vi "4Pi DCM - Crop Image.vi"(9 "ROI Size":i32=3, 10 "Image Refs":T1[](array[typedef]), 11 "Input Image (U16)":u16[][](array[numeric])) -> (3 "Output Image Stack":u16[][][](array[numeric]))   [LabVIEW 2016]
uses:
  <vilib>/vision/Image Controls.llb/IMAQ Image.ctl
  Display Module/Display Module Custom Controls/ROI Descriptor.ctl
panel:
  out "ROI4":u16[][](graph)
  out "ROI3":u16[][](graph)
  out "ROI2":u16[][](graph)
  out "ROI1":u16[][](graph)
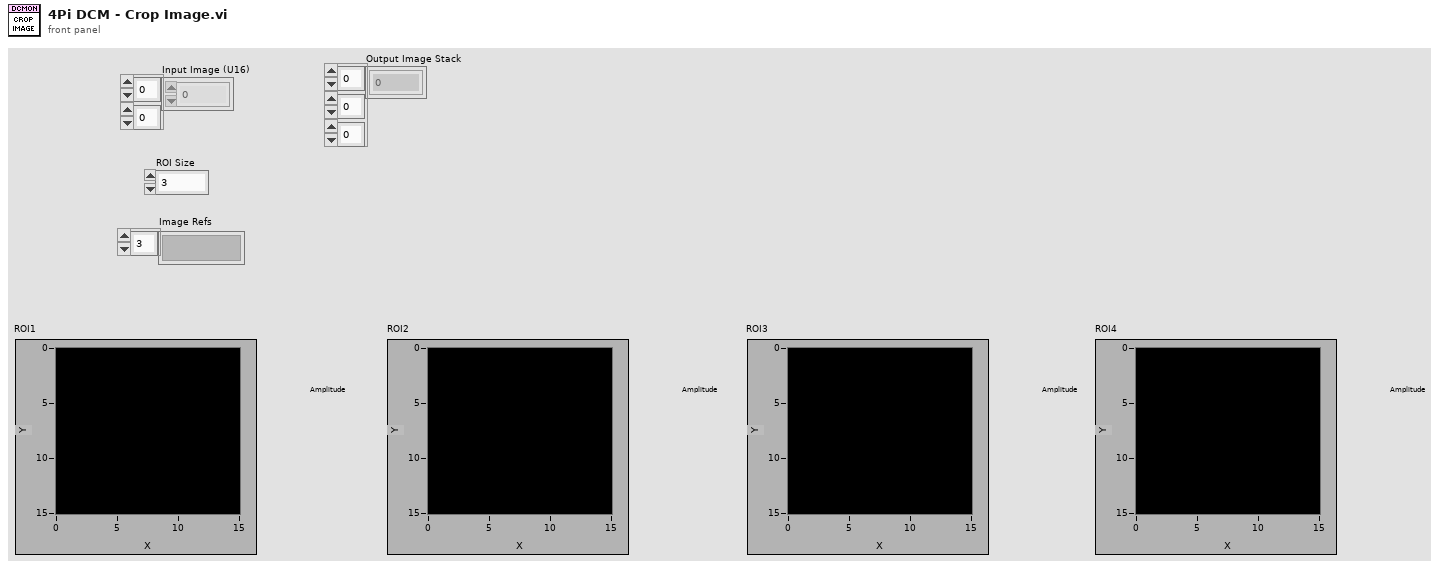
[diagram p1: front panel]
types:
  T1 = typedef "IMAQ Image.ctl" = refnum<image>
  T2 = typedef "ROI Descriptor.ctl" = cluster{"Global Rectangle":i32[], "Contours":cluster{"Contour Type":u32, "ROI Type":u32, "Points":i32[]}[]}
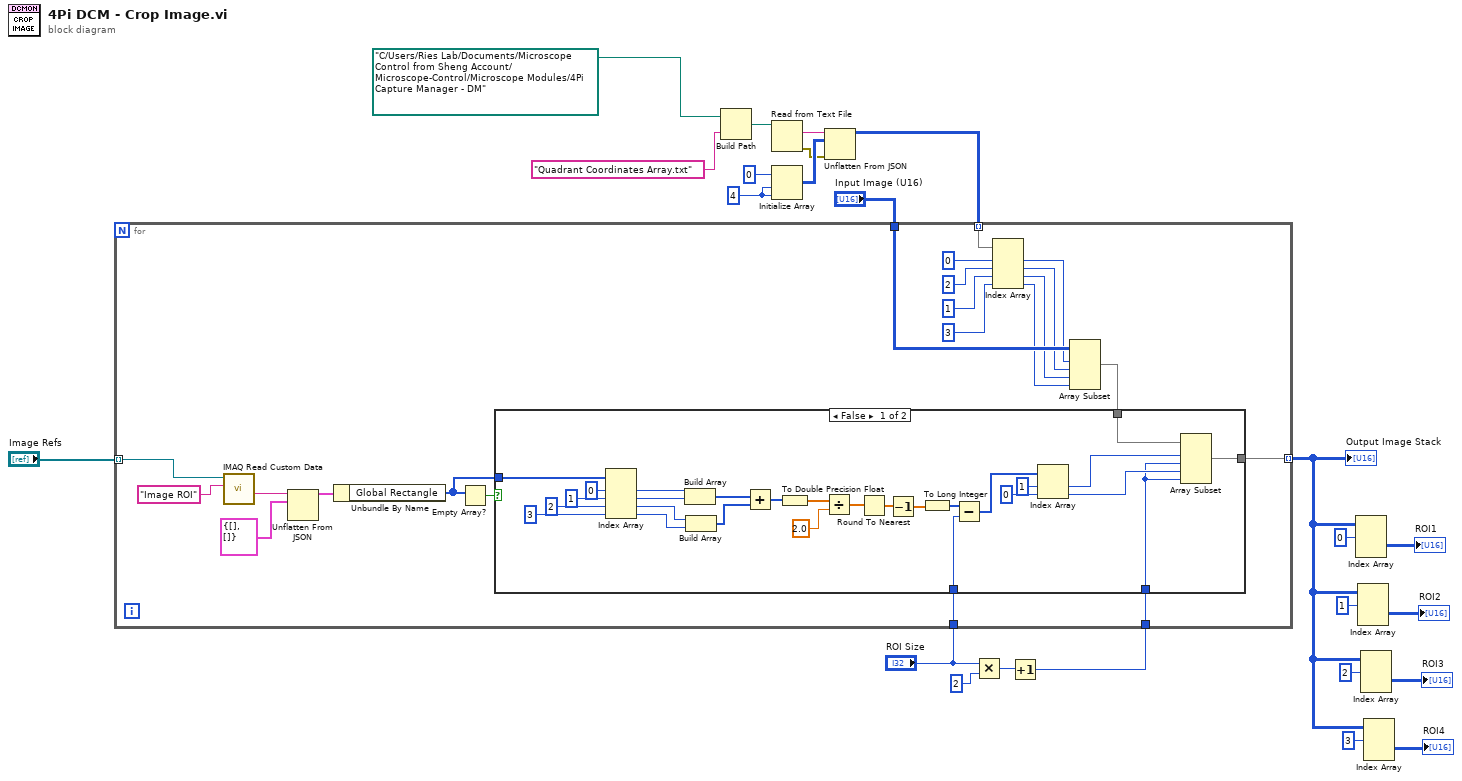
[diagram p0: block diagram]
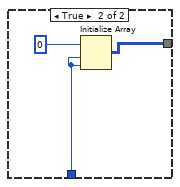
[diagram p2: hidden frame]
diagram:
  w18 = 4 ("dimension size")
  n1 = Build Path(base path=path "C:/Users/Ries Lab/Documents/Microscope Control from Sheng Account/Microscope-Control/Microscope Modules/4Pi Capture Manager - DM" ("path"), name or relative path="Quadrant Coordinates Array.txt") -> (appended path=w21:path)
  n2 = Read from Text File(file (use dialog)=w21) -> (text=w20:string, error out=w19:errorcluster)  [unwired: 3 in, 2 out]
  n3 = Initialize Array(0 ("element"), w18, w18) -> (w22:i32[][])
  n4 = Unflatten From JSON(JSON string=w20, type and defaults=w22, error in (no error)=w19) -> (value=w17:i32[][])  [unwired: 4 in, 1 out]
  n5 = Multiply(x="ROI Size", y=2) -> (x*y=w14:i32)
  n6 = Increment(x=w14) -> (x+1=w13:i32)
  n7 = for {
    tunnel: w17 -> [w45] mode=indexing
    tunnel: "Input Image (U16)" -> [w44]
    tunnel: w13 -> [w28]
    tunnel: "ROI Size" -> [w27]
    tunnel: [w26] -> w2 mode=indexing
    tunnel: "Image Refs" -> [w25] mode=indexing
    n8 = call "IMAQ Read Custom Data"("Key"="Image ROI", "Image"=w25) -> ("Custom Data Out"=w33:string)  [unwired: 7 in, 2 out]
    n9 = Unflatten From JSON(JSON string=w33, type and defaults=T2 {"Global Rectangle"=[], "Contours"=[]} ("Image ROI Descriptor")) -> (value=w31:T2)  [unwired: 5 in, 1 out]
    n10 = Unbundle By Name(w31) -> ("Global Rectangle"=w29:i32[])
    n11 = Empty Array?(array=w29) -> (empty?=w30:bool)
    n12 = Index Array(array=w45, index #1=0 ("index"), index #2=2 ("index"), index #3=1 ("index"), index #4=3 ("index")) -> (element #1=w42:i32, element #2=w41:i32, element #3=w37:i32, element #4=w36:i32)
    n13 = Array Subset(array=w44, index (row)=w42, length (row)=w41, index (col)=w37, length (col)=w36) -> (w35:u16[][])
    n14 = case shown="False" w30 {
      tunnel: w35 -> [w52 _]
      tunnel: [w51 w73] -> w26
      tunnel: w29 -> [w50 _]
      tunnel: w28 -> [w49 w74]
      tunnel: w27 -> [w48 _]
      frame False {
        n15 = Index Array(array=w50, index #1=0 ("index"), index #2=1 ("index"), index #3=2 ("index"), index #4=3 ("index")) -> (element #1=w65:i32, element #2=w64:i32, element #3=w63:i32, element #4=w62:i32)
        n16 = Build Array(w65, w64) -> (w61:i32[])
        n17 = Build Array(w63, w62) -> (w60:i32[])
        n18 = Add(x=w61, y=w60) -> (x+y=w67:i32[])
        n19 = To Double Precision Float(number=w67) -> (double precision float=w68:dbl[])
        n20 = Divide(x=w68, y=2.0) -> (x/y=w59:dbl[])
        n21 = Round To Nearest(number=w59) -> (nearest integer value=w47:dbl[])
        n22 = Decrement(x=w47) -> (x-1=w46:dbl[])
        n23 = To Long Integer(number=w46) -> (32bit integer=w58:i32[])
        n24 = Subtract(x=w58, y=w48) -> (x-y=w57:i32[])
        n25 = Index Array(array=w57, index #1=1 ("index"), index #2=0 ("index")) -> (element #1=w54:i32, element #2=w53:i32)
        n26 = Array Subset(array=w52, index (row)=w54, length (row)=w49, index (col)=w53, length (col)=w49) -> (w51:u16[][])
      }
      frame True {
        n27 = Initialize Array(u16 0, w74, w74) -> (w73:u16[][])
      }
    }
  }
  "Output Image Stack" <- w2
  n28 = Index Array(array=w2, index (dim 0)=0 ("index (page)")) -> (element=→"ROI1":u16[][])  [unwired: 2 in]
  n29 = Index Array(array=w2, index (dim 0)=1 ("index (page)")) -> (element=→"ROI2":u16[][])  [unwired: 2 in]
  n30 = Index Array(array=w2, index (dim 0)=2 ("index (page)")) -> (element=→"ROI3":u16[][])  [unwired: 2 in]
  n31 = Index Array(array=w2, index (dim 0)=3 ("index (page)")) -> (element=→"ROI4":u16[][])  [unwired: 2 in]
